vi "Requests.vi"(8 "error in (no error)":errorcluster, 9 "write enable":bool=TRUE, 11 "OHAUS in":refnum<class "OHAUS_Navigator.lvclass">) -> (0 "error out":errorcluster, 3 "OHAUS out":refnum<class "OHAUS_Navigator.lvclass">)   [LabVIEW 2019, in "OHAUS_Navigator.lvclass"]
uses:
  OHAUS_Navigator.lvclass
  C:/my_projects/projects/Algorithms/Labview/19/Modbus/MB_TCP2/MB_TCP.lvclass
  MB_TCP.lvclass/MB_TCP.ctl
  NI_modbus_upd/TCP/TCP.lvclass/TCP.ctl
  <vilib>/Utility/error.llb/Clear Errors.vi
  NI_modbus_upd/TCP/TCP.lvclass
  ICPCON Registers/ICPCON Registers.lvlib
  MB_TCP.lvclass
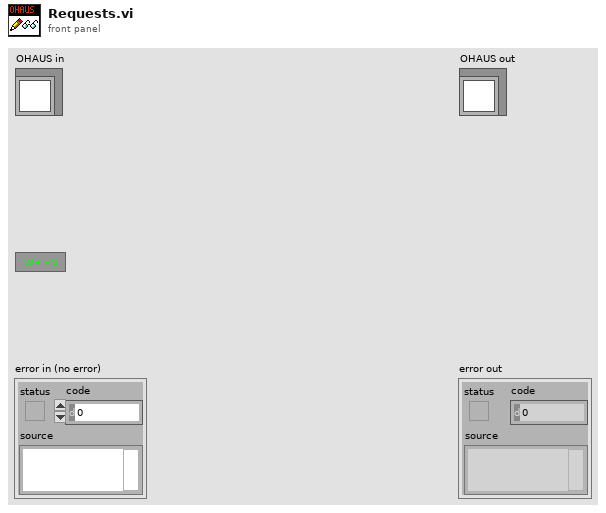
[diagram p1: front panel]
types:
  T1 = enum16{"Standard", "Buffered", "CRLF", "Immediate"}
  T2 = typedef "ICPCON Registers.lvlib/ICPCON Data.ctl" = cluster{"UTF":refnum<data-value>, "DI":refnum<data-value>, "DW":refnum<data-value>, "DO":refnum<data-value>, "IR":refnum<data-value>, "WR":refnum<data-value>, "OR":refnum<data-value>, "modified":refnum<data-value>}
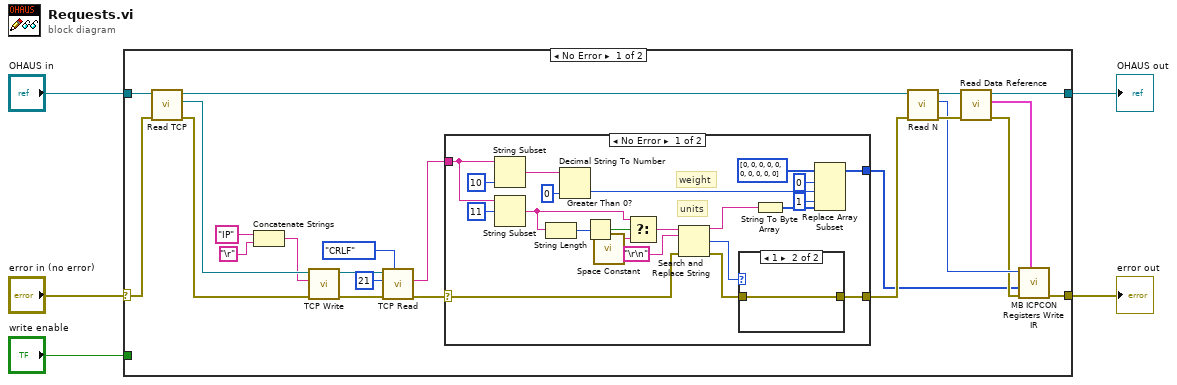
[diagram p0: block diagram]
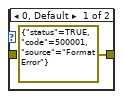
[diagram p2: hidden frame]
diagram:
  n1 = case shown="No Error" "error in (no error)" {
    selector: "error in (no error)" -> [w24 w55]
    tunnel: [w6 w55] -> w3
    tunnel: [w22 w54] -> w4
    tunnel: "OHAUS in" -> [w25 w54]
    tunnel: "write enable" -> [_ _]
    frame No Error {
      n2 = call "Read TCP.vi"("error in (no error)"=w24, "MB_TCP in"=w25) -> ("error out"=w18:errorcluster, "TCP"=w19:refnum<class "TCP.lvclass">, "MB_TCP out"=w23:refnum<class "OHAUS_Navigator.lvclass">)  [unwired: 7 in]
      n3 = Concatenate Strings("IP" ("Code"), "\r") -> (w15:string)
      n4 = call "TCP Write.vi"("error in (no error)"=w18, "data"=w15, "protocol layer in"=w19) -> ("error out"=w12:errorcluster, "protocol layer out"=w14:refnum<class "TCP.lvclass">)  [unwired: 6 in, 1 out]
      n5 = call "TCP Read.vi"("mode (standard)"=T1."CRLF", "error in (no error)"=w12, "bytes to read"=21, "TCP in"=w14) -> ("error out"=w10:errorcluster, "data"=w9:string)  [unwired: 4 in, 2 out]
      n6 = case shown="No Error" w10 {
        selector: w10 -> [w32 w53]
        tunnel: w9 -> [w46 _]
        tunnel: [w30 w53] -> w8
        tunnel: [w37 _] -> w7
        frame No Error {
          # "units"
          # "weight"
          n7 = String Subset(string=w46, length (rest)=10 ("length (rest)")) -> (substring=w48:string)  [unwired: 1 in]
          n8 = String Subset(string=w46, offset (0)=11 ("length (rest)")) -> (substring=w44:string)  [unwired: 1 in]
          n9 = String Length(string=w44) -> (length=w36:i32)
          n10 = Decimal String To Number(string=w48, default (0L)=0 ("default (0 I32)")) -> (number=w38:i32)  [unwired: 1 in, 1 out]
          n11 = Greater Than 0?(x=w36) -> (x > 0?=w45:bool)
          n12 = call <vilib>:"Space Constant.vi"() -> ("String"=w43:string)
          n13 = Select(t=w44, s=w45, f=w43) -> (s? t:f=w35:string)
          n14 = Search and Replace String(input string=w35, search string="\r\n", error in=w32) -> (result string=w34:string, number of replacements=w31:i32, error out=w29:errorcluster)  [unwired: 5 in, 1 out]
          n15 = case shown="1" w31 {
            tunnel: [errorcluster {"status"=TRUE, "code"=500001, "source"="Format Error"} ("error IO") w52] -> w30
            tunnel: w29 -> [_ w52]
            frame 0, Default {
            }
            frame 1 {
            }
          }
          n16 = String To Byte Array(string=w34) -> (unsigned byte array=w39:u8[])
          n17 = Replace Array Subset(array=u16[] [0, 0, 0, 0, 0, 0, 0, 0, 0, 0] ("Registers"), new element #1=w38, index #1=0 ("index"), new element #2=w39, index #2=1 ("index")) -> (w37:u16[])
        }
        frame Error {
        }
      }
      n18 = call "Read N.vi"("error in (no error)"=w8, "MB_TCP in"=w23) -> ("error out"=w28:errorcluster, "N"=w21:i32, "MB_TCP out"=w27:refnum<class "OHAUS_Navigator.lvclass">)  [unwired: 7 in]
      n19 = call "Read Data Reference.vi"("error in (no error)"=w28, "MB_TCP in"=w27) -> ("error out"=w20:errorcluster, "Data"=w26:T2, "MB_TCP out"=w22:refnum<class "OHAUS_Navigator.lvclass">)  [unwired: 7 in]
      n20 = call "MB ICPCON Registers Write IR.vi"("Data Reference"=w26, "error in (no error)"=w20, "Words In"=w7, "N"=w21) -> ("error out"=w6:errorcluster)  [unwired: 7 in]
    }
    frame Error {
    }
  }
  "error out" <- w3
  "OHAUS out" <- w4
